vi "measure.vi"() -> ()   [LabVIEW 2015]
uses:
  <vilib>/gmath/SpecialFunctions.llb/Factorial.vi
  <vilib>/Utility/file.llb/Read Delimited Spreadsheet (DBL).vi
  <vilib>/Utility/file.llb/Read Delimited Spreadsheet (I64).vi
  <vilib>/imath/engines/lvmath2/RunTimeEngine/Managers/WorkSpace/UID Generator.vi
  <vilib>/imath/engines/lvmath2/RunTimeEngine/RunTimeType/NIMS_RunTimeType_From StrictType (excl LVString).vi
  <instcachedir>/0/NIMS_RunTimeType_From StrictType (excl LVString)_EB1C38A9BC5048DA9ABDA8F781E54D21.lvgen/NIMS_RunTimeType_From StrictType (excl LVString)_EB1C38A9BC5048DA9ABDA8F781E54D21_000.vi
  <vilib>/imath/engines/lvmath2/RunTimeEngine/LocalVariableDefStatement/MC_LocalVariableDefStatement_Display.vi
  <vilib>/imath/engines/lvmath2/RunTimeEngine/ArithmeticOperatorToken/NIMS_ArithmeticOperator_rightdiv.vi
  <instcachedir>/0/NIMS_ArithmeticOperator_rightdiv_E8FF7CD3D5774FA6AA728C3F0517CAD4.lvgen/NIMS_ArithmeticOperator_rightdiv_E8FF7CD3D5774FA6AA728C3F0517CAD4_000.vi
  <vilib>/imathl/engines/lvmath/Functions/Error Handling/Create Error.vi
  <vilib>/imath/engines/lvmath2/RunTimeEngine/Managers/SymbolTable/Clear UID.vi
  <vilib>/imath/engines/lvmath2/RunTimeEngine/NodeEndStatement/NIMS_NodeEndStatement_Output.vi
  <instcachedir>/0/NIMS_NodeEndStatement_Output_53EC0D466D134D7ABD903AC30B43404B.lvgen/NIMS_NodeEndStatement_Output_53EC0D466D134D7ABD903AC30B43404B_011.vi
  <instcachedir>/0/NIMS_NodeEndStatement_Output_53EC0D466D134D7ABD903AC30B43404B.lvgen/NIMS_NodeEndStatement_Output_53EC0D466D134D7ABD903AC30B43404B_005.vi
  <vilib>/imath/engines/lvmath2/RunTimeEngine/ErrorHandling/NIMS_Finalize Error.vi
  <vilib>/Analysis/NI_AALBase.lvlib
  <vilib>/gmath/NI_Gmath.lvlib
  <vilib>/imath/engines/lvmath2/RunTimeEngine/Managers/SymbolTable/NIMS_WorkSpace.lvlib
panel:
  out "Decay Rate [s]":dbl=186.38316419739238
  out "Constant Rate":cluster{"X Values":dbl[], "f":dbl[]}[](graph)=[{"X Values"=[0.5666666666666667, 1.7, 2.8333333333333335, 3.966666666666667, 5.1, 6.233333333333333, 7.366666666666666, 8.5, 9.633333333333333, 10.766666666666667, 11.9, 13.033333333333333, 14.166666666666666, 15.3, 16.433333333333334, 17.566666666666666, 18.7, 19.833333333333332, 20.966666666666665, 22.1, 23.233333333333334, 24.366666666666667, 25.5, 26.633333333333333, 27.766666666666666, 28.9, 30.033333333333335, 31.166666666666668, 32.3, 33.43333333333333, 34.56666666666667, 35.7, 36.833333333333336, 37.96666666666667, 39.1, 40.233333333333334, 41.36666666666667, 42.5, 43.63333333333333, 44.766666666666666, 45.9, 47.03333333333333, 48.166666666666664, 49.3, 50.43333333333333, 51.56666666666667, 52.7, 53.833333333333336, 54.96666666666667, 56.1, 57.233333333333334, 58.36666666666667, 59.5, 60.63333333333333, 61.766666666666666, 62.9, 64.03333333333333, 65.16666666666667, 66.3, 67.43333333333334], "f"=[1.0, 0.0, 0.0, 0.0, 0.0, 0.0, 0.0, 0.0, 0.0, 0.0, 0.0, 0.0, 0.0, 0.0, 0.0, 0.0, 0.0, 0.0, 0.0, 0.0, 0.0, 0.0, 0.0, 0.0, 0.0, 0.0, 1.0, 1.0, 1.0, 1.0, 2.0, 0.0, 1.0, 2.0, 5.0, 5.0, 4.0, 17.0, 7.0, 2.0, 10.0, 10.0, 7.0, 8.0, 7.0, 10.0, 2.0, 3.0, 3.0, 0.0, 2.0, 2.0, 2.0, 2.0, 2.0, 0.0, 0.0, 0.0, 0.0, 1.0]}, {"X Values"=[0.0, 1.0, 2.0, 3.0, 4.0, 5.0, 6.0, 7.0, 8.0, 9.0, 10.0, 11.0, 12.0, 13.0, 14.0, 15.0, 16.0, 17.0, 18.0, 19.0, 20.0, 21.0, 22.0, 23.0, 24.0, 25.0, 26.0, 27.0, 28.0, 29.0, 30.0, 31.0, 32.0, 33.0, 34.0, 35.0, 36.0, 37.0, 38.0, 39.0, 40.0, 41.0, 42.0, 43.0, 44.0, 45.0, 46.0, 47.0, 48.0, 49.0, 50.0, 51.0, 52.0, 53.0, 54.0, 55.0, 56.0, 57.0, 58.0, 59.0, 60.0, 61.0, 62.0, 63.0, 64.0, 65.0, 66.0, 67.0, 68.0, 69.0, 70.0, 71.0, 72.0, 73.0, 74.0, 75.0, 76.0, 77.0, 78.0, 79.0, 80.0, 81.0, 82.0, 83.0, 84.0, 85.0, 86.0, 87.0, 88.0, 89.0, 90.0, 91.0, 92.0, 93.0, 94.0, 95.0, 96.0, 97.0, 98.0, 99.0, 100.0, 101.0, 102.0, 103.0, 104.0, 105.0, 106.0, 107.0, 108.0, 109.0, 110.0, 111.0, 112.0, 113.0, 114.0, 115.0, 116.0, 117.0, 118.0, 119.0, 120.0], "f"=[2.565295348933683e-19, 1.231341767488168e-17, 2.9552202419716033e-16, 4.728352387154565e-15, 5.674022864585479e-14, 5.447061950002059e-13, 4.357649560001647e-12, 2.9881025554297006e-11, 1.7928615332578206e-10, 9.561928177375042e-10, 4.589725525140021e-09, 2.0027893200610997e-08, 8.011157280244399e-08, 2.9579657650133165e-07, 1.0141596908617085e-06, 3.245311010757468e-06, 9.735933032272402e-06, 2.748969326759267e-05, 7.330584871358044e-05, 0.00018519372306588744, 0.00044446493535812986, 0.0010159198522471538, 0.002216552404902881, 0.004625848497188621, 0.009251696994377244, 0.01776325822920431, 0.03279370750006949, 0.05829992444456798, 0.0999427276192594, 0.16542244571463624, 0.26467591314341804, 0.4098207687381956, 0.6147311531072934, 0.8941544045196996, 1.262335629910164, 1.7312031495910822, 2.3082708661214433, 2.9945135560494403, 3.782543439220344, 4.655438079040424, 5.5865256948485085, 6.540322764700694, 7.474654588229364, 8.343800470581614, 9.102327786089035, 9.709149638494969, 10.1312865792991, 10.346845868220356, 10.346845868220358, 10.135685748460759, 9.73025831852233, 9.15789018213866, 8.453437091204917, 7.6559430259969075, 6.805282689775029, 5.939155801985478, 5.09070497313041, 4.286909451057188, 3.5477871319093968, 2.8863352937567974, 2.3090682350054372, 1.8169717259059184, 1.4066877877981303, 1.0717621240366706, 0.8038215930275031, 0.5935913302356948, 0.4317027856259596, 0.3092796076126279, 0.21831501713832552, 0.15187131627013947, 0.1041403311566671, 0.07040473092281717, 0.0469364872818781, 0.03086234780178287, 0.020018820195751054, 0.012812044925280678, 0.00809181784754569, 0.005044250086781729, 0.0031041538995579864, 0.0018860681921364982, 0.0011316409152818988, 0.0006706020238707549, 0.0003925475261682468, 0.00022701543682019092, 0.0001297231067543948, 7.32554014613053e-05, 4.0886735699333195e-05, 2.2558199006528653e-05, 1.2304472185379268e-05, 6.636119830316909e-06, 3.5392639095023507e-06, 1.8668644797375036e-06, 9.74016250297828e-07, 5.027180646698467e-07, 2.567070968526877e-07, 1.2970463840977905e-07, 6.485231920488952e-08, 3.2091869297264924e-08, 1.571846659457874e-08, 7.621074712523023e-09, 3.6581158620110514e-09, 1.7385105086785192e-09, 8.181225923193032e-10, 3.812610138963744e-10, 1.7596662179832664e-10, 8.04418842506636e-11, 3.642651362294201e-11, 1.6340865924310432e-11, 7.262607077471305e-12, 3.198212290996537e-12, 1.3955835451621256e-12, 6.034955870971353e-13, 2.5864096589877224e-13, 1.0986518905434578e-13, 4.625902697025084e-14, 1.930811560497426e-14, 7.989565077920385e-15, 3.277770288377594e-15, 1.3333302867976654e-15, 5.37813897195697e-16, 2.1512555887827878e-16]}]
  out "Decay Plot":dbl[][](graph)=[[0.0, 62.0, 62.0, 72.0, 42.0, 37.0, 40.0, 36.0, 44.0, 36.0, 43.0, 42.0, 29.0, 39.0, 49.0, 46.0, 31.0, 36.0, 31.0, 30.0, 39.0, 34.0, 41.0, 31.0, 35.0, 30.0, 32.0, 25.0, 31.0, 35.0, 27.0, 29.0, 29.0, 29.0, 32.0, 34.0, 27.0, 26.0, 27.0, 27.0, 29.0, 34.0, 28.0, 31.0, 27.0, 24.0, 28.0, 25.0, 27.0, 32.0, 18.0, 19.0, 39.0, 21.0, 26.0, 19.0, 22.0, 32.0, 20.0, 22.0, 26.0, 19.0, 21.0, 22.0, 23.0, 20.0, 29.0, 24.0, 15.0, 23.0, 25.0, 19.0, 20.0, 20.0, 23.0, 18.0, 15.0, 22.0, 13.0, 14.0, 21.0, 21.0, 26.0, 11.0, 10.0, 17.0, 17.0, 21.0, 13.0, 16.0, 13.0, 18.0, 14.0, 17.0, 16.0, 17.0, 13.0, 5.0, 14.0, 12.0, 15.0, 21.0, 14.0, 18.0, 18.0, 9.0, 22.0, 23.0, 11.0, 16.0, 14.0, 13.0, 9.0, 10.0, 16.0, 19.0, 15.0, 7.0, 8.0, 10.0, 7.0, 18.0, 9.0, 8.0, 20.0, 9.0, 9.0, 9.0, 10.0, 10.0, 10.0, 17.0, 12.0, 10.0, 10.0, 12.0, 9.0, 6.0, 6.0, 11.0, 13.0, 9.0, 8.0, 11.0, 7.0, 12.0, 9.0, 6.0, 10.0, 9.0, 11.0, 9.0, 6.0, 8.0, 10.0, 9.0, 6.0, 8.0, 6.0, 12.0, 12.0, 11.0, 14.0, 8.0, 10.0, 8.0, 7.0, 13.0, 11.0, 7.0, 9.0, 8.0, 10.0, 7.0, 7.0, 7.0, 7.0, 7.0, 4.0, 9.0, 8.0, 10.0, 6.0, 10.0, 7.0, 10.0, 5.0, 7.0, 5.0, 8.0, 6.0, 4.0, 6.0, 1.0, 9.0, 2.0, 3.0, 5.0, 6.0, 7.0, 5.0, 8.0, 4.0, 9.0, 5.0, 8.0, 7.0, 5.0, 6.0, 4.0, 6.0, 3.0, 3.0, 8.0, 8.0, 5.0, 3.0, 5.0, 7.0, 3.0, 6.0, 2.0, 4.0, 6.0, 3.0, 3.0, 5.0, 4.0, 3.0, 6.0, 6.0, 8.0, 4.0, 7.0, 6.0, 8.0, 6.0, 7.0, 8.0, 2.0], [56.17689860571011, 37.04230741987081, 36.782872262499374, 36.52482532293666, 36.26815917293469, 36.01286642399346, 35.75893972714829, 35.50637177275823, 35.255155290295676, 35.00528304813708, 34.75674785335472, 34.50954255150972, 34.263660026446054, 34.01909320008569, 33.775835032224876, 33.53387852033145, 33.293216699343255, 33.05384264146767, 32.81574945598213, 32.57893028903586, 32.34337832345247, 32.109086778533786, 31.876048909864636, 31.644258009118673, 31.413707403865338, 31.184390457377717, 30.956300568441506, 30.729431171165018, 30.503775734790146, 30.27932776350437, 30.056080796253767, 29.834028406557046, 29.613164202320483, 29.393481825654007, 29.174974952688117, 28.957637293391834, 28.74146259139171, 28.52644462379162, 28.312577200993708, 28.099854166520196, 27.88826939683613, 27.67781680117315, 27.468490321354096, 27.2602839316187, 27.053191638450045, 26.847207480402083, 26.642325527928, 26.438539883209565, 26.23584467998728, 26.034234083391574, 25.83370228977485, 25.634243526544346, 25.435852051996008, 25.23852215514924, 25.042248155582442, 24.8470244032695, 24.652845278417217, 24.459705191303428, 24.267598582116165, 24.076519920793594, 23.88646370686483, 23.697424469291576, 23.509396766310637, 23.322375185277302, 23.1363543425095, 22.951328883132838, 22.767293480926426, 22.584242838169615, 22.402171685489428, 22.221074781708907, 22.040946913696246, 21.8617828962147, 21.683577571773327, 21.506325810478543, 21.330022509886433, 21.15466259485585, 20.980241017402356, 20.80675275655291, 20.634192818201292, 20.462556234964367, 20.2918380660391, 20.12203339706032, 19.953137339959238, 19.785145032822754, 19.618051639753503, 19.451852350730626, 19.28654238147133, 19.122116973293153, 18.95857139297699, 18.795900932630804, 18.63410090955416, 18.473166666103392, 18.313093569557516, 18.1538770119849, 17.995512410110592, 17.83799520518442, 17.681320862849702, 17.52548487301278, 17.37048274971316, 17.216310030994382, 17.062962278775565, 16.910435078723673, 16.758724040126427, 16.607824795765914, 16.45773300179287, 16.308444337601653, 16.159954505705834, 16.012259231614518, 15.865354263709278, 15.71923537312179, 15.573898353612066, 15.429339021447394, 15.285553215281901, 15.142536796036758, 15.00028564678103, 14.858795672613166, 14.71806280054313, 14.57808297937514, 14.438852179591041, 14.300366393234356, 14.16262163379485, 14.025613936093809, 13.889339356169895, 13.753793971165603, 13.61897387921434, 13.484875199328101, 13.351494071285764, 13.218826655521948, 13.086869133016492, 12.955617705184533, 12.825068593767131, 12.695218040722537, 12.566062308117996, 12.437597678022133, 12.309820452397958, 12.182726952996394, 12.056313521250374, 11.930576518169573, 11.805512324235622, 11.681117339297899, 11.557387982469937, 11.434320692026315, 11.31191192530012, 11.190158158580996, 11.06905588701369, 10.948601624497158, 10.828791903584229, 10.709623275381762, 10.59109230945139, 10.47319559371077, 10.35592973433533, 10.239291355660619, 10.123277100085094, 10.007883627973484, 9.89310761756066, 9.778945764856008, 9.665394783548301, 9.552451404911132, 9.440112377708783, 9.328374468102663, 9.21723445955821, 9.106689152752274, 8.996735365481062, 8.8873699325685, 8.778589705775126, 8.670391553707482, 8.562772361727955, 8.455729031865108, 8.349258482724522, 8.243357649400103, 8.138023483385798, 8.033252952487913, 7.929043040737781, 7.825390748304944, 7.722293091410826, 7.619747102242805, 7.5177498288688085, 7.416298335152337, 7.315389700667918, 7.2150210206170655, 7.1151894057446405, 7.015891982255692, 6.917125891732731, 6.818888291053444, 6.721176352308834, 6.623987262721858, 6.5273182245664, 6.431166455086778, 6.335529186417627, 6.2404036655042106, 6.145787154023182, 6.051676928303767, 5.95807027924932, 5.864964512259391, 5.772356947152122, 5.6802449180871015, 5.58862577348863, 5.497496875969393, 5.406855602254524, 5.316699343106112, 5.227025503248079, 5.137831501291462, 5.049114769660125, 4.960872754516828, 4.873102915689728, 4.785802726599247, 4.6989696741853315, 4.612601258835134, 4.526694994311052, 4.441248407679122, 4.356259039237894, 4.271724442447578, 4.18764218385963, 4.1040098430467165, 4.020825012533015, 3.9380852977249248, 3.8557883168421405, 3.7739317008490794, 3.6925130933866797, 3.611530150704592, 3.5309805415936832, 3.4508619473189537, 3.371172061552775, 3.2919085903084984, 3.213069251874428, 3.134651776748134, 3.0566539075711177, 2.9790733990638394, 2.9019080179610786, 2.825155542947636, 2.7488137645944217, 2.6728804852948187, 2.597353519201434, 2.5222306921631894, 2.447509841662713, 2.373188816754105, 2.299265478001015, 2.2257376974150453, 2.1526033583945114, 2.0798603556635022]]
  in  "Decay Measurement":path=path "C:/Users/mohamm2/Desktop/week8sd/keaton2.txt"
  in  "Constant Rate Measurement":path=path "C:/Users/mohamm2/Desktop/week8sd/uranium2.txt"
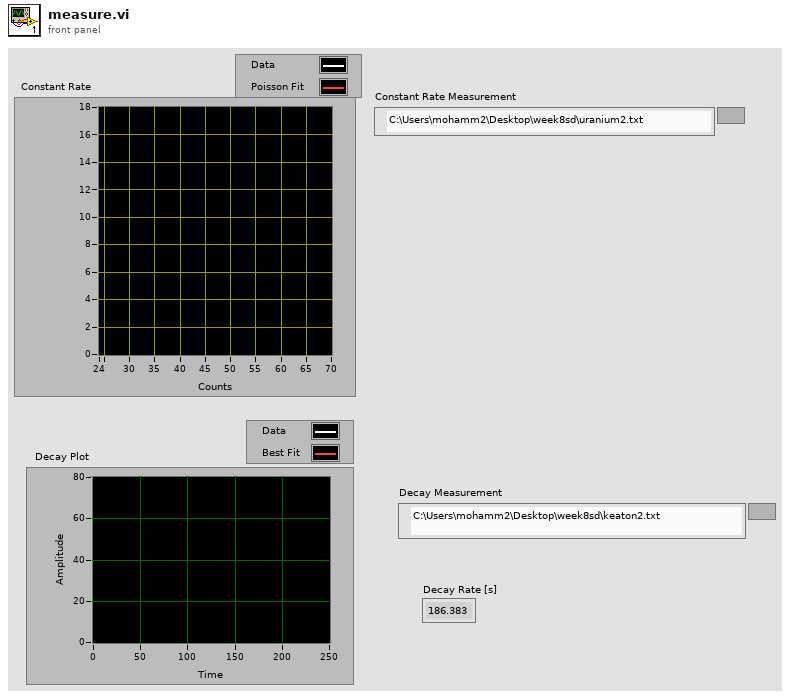
[diagram p1: front panel]
types:
  T1 = cluster{"Array[0]":dbl, "Array[1]":dbl, "Array[2]":dbl, "Array[3]":dbl, "Array[4]":dbl, "Array[5]":dbl, "Array[6]":dbl, "Array[7]":dbl, "Array[8]":dbl}
  T2 = cluster{"X Values":dbl[], "Histogram: h(x)":i32[]}
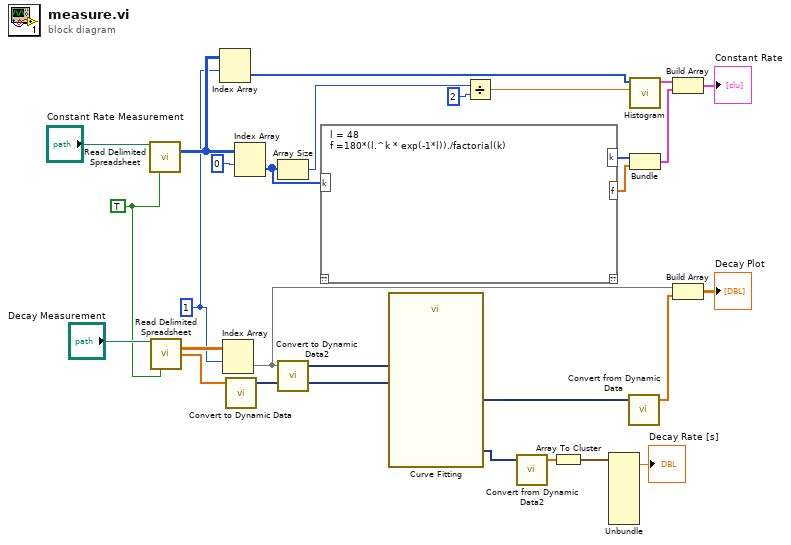
[diagram p0: block diagram]
diagram:
  w21 = 1
  w26 = TRUE
  n1 = call-poly <vilib>:"Read Delimited Spreadsheet.vi"("file path (dialog if empty)"="Constant Rate Measurement", "transpose? (F)"=w26) -> ("all rows"=w24:i64[][])  [unwired: 8 in, 5 out]
  n2 = call-poly <vilib>:"Read Delimited Spreadsheet.vi"("file path (dialog if empty)"="Decay Measurement", "transpose? (F)"=w26) -> ("all rows"=w22:dbl[][], "first row"=w20:dbl[])  [unwired: 8 in, 4 out]
  n3 = Index Array(array=w24, index (row)=w21) -> (element=w23:i64[])  [unwired: 1 in]
  n4 = Index Array(array=w22, index (row)=w21) -> (element=w5:dbl[])  [unwired: 1 in]
  n5 = call "Convert to Dynamic Data"("Array"=w20) -> ("Dynamic Data Type"=w19:dynamicdata)  [unwired: 3 in]
  n6 = Index Array(array=w24, index (row)=0) -> (element=w9:i64[])  [unwired: 1 in]
  n7 = Array Size(array=w9) -> (size(s)=w10:i32)
  n8 = call "Convert to Dynamic Data2"("Array"=w5) -> ("Dynamic Data Type"=w18:dynamicdata)  [unwired: 3 in]
  n9 = mathscript code="l = 48\nf =180*(l.^k * exp(-1*l))./factorial(k)"("k"=w9) -> ("f"=w7:dbl[], "k"=w8:i64[])  [unwired: 1 in, 1 out]
  n10 = call "Curve Fitting"("Locations"=w19, "Signals"=w18) -> ("best fit"=w16:dynamicdata, "non-linear coefficients"=w4:dynamicdata)  [unwired: 5 in, 3 out]
  n11 = Divide(x=w10, y=2) -> (x/y=w11:dbl)
  n12 = call "Convert from Dynamic Data2"("Dynamic Data Type"=w4) -> ("Array"=w3:dbl[])  [unwired: 3 in]
  n13 = Array To Cluster(array=w3) -> (cluster=w2:T1)
  n14 = Unbundle(w2) -> ("Array[1]"=→"Decay Rate [s]":dbl)  [unwired: 8 out]
  n15 = call "Convert from Dynamic Data"("Dynamic Data Type"=w16) -> ("Array"=w15:dbl[])  [unwired: 3 in]
  n16 = call <vilib>:"Histogram.vi"("intervals"=w11, "X"=w23) -> ("Histogram Graph"=w14:T2)  [unwired: 6 in, 3 out]
  n17 = Bundle("k"=w8, "f"=w7) -> (w6:cluster{"k":i64[], "f":dbl[]})  [unwired: 1 in]
  n18 = Build Array(w14, w6) -> (→"Constant Rate":cluster{"X Values":dbl[], "f":dbl[]}[])
  n19 = Build Array(w5, w15) -> (→"Decay Plot":dbl[][])
